vi "thermo_close.vi"(8 "error in":errorcluster, 11 "thermo in":T1={"type"=enum."COMET Tx5xx (ethernet)", "comment"="", "tag"="", "refresh"=0.0, "IP"="", "port"=0, "VISA"="", "last readout"=timestamp(0 s since 1904-01-01), "TCP ref"=refnum, "VISA sess"="", "idn"="", "press"=0.0, "RH"=0.0, "temp"=0.0, "pres cor"=[], "RH cor"=[], "temp cor"=[], "try left"=0, "failed"=FALSE, "RTD set"=[], "RTD inv"=[], "range"=0.0, "net mode"=enum."MODBUS", "try fail"=enum."Stop trying - return NaN", "timeout [s]"=0.0, "max retries"=0, "sim t [deg]"=0.0} {"RTD inv" format="%.1f"; "RTD set" format="%.1f"; "temp cor" format="%.1f"; "RH cor" format="%.1f"; "pres cor" format="%.1f"; "refresh" min=0.1 max=1000.0 format="%.2f"}) -> (0 "error out":errorcluster, 3 "thermo out":T1={"type"=enum."COMET Tx5xx (ethernet)", "comment"="", "tag"="", "refresh"=0.0, "IP"="", "port"=0, "VISA"="", "last readout"=timestamp(0 s since 1904-01-01), "TCP ref"=refnum, "VISA sess"="", "idn"="", "press"=0.0, "RH"=0.0, "temp"=0.0, "pres cor"=[], "RH cor"=[], "temp cor"=[], "try left"=0, "failed"=FALSE, "RTD set"=[], "RTD inv"=[], "range"=0.0, "net mode"=enum."MODBUS", "try fail"=enum."Stop trying - return NaN", "timeout [s]"=0.0, "max retries"=0, "sim t [deg]"=0.0} {"RTD inv" format="%.1f"; "RTD set" format="%.1f"; "temp cor" format="%.1f"; "RH cor" format="%.1f"; "pres cor" format="%.1f"; "refresh" min=0.1 max=1000.0 format="%.2f"})   [LabVIEW 2020]
uses:
  thermo.ctl
  thermo_types.ctl
  Thermometer Fail Action.ctl
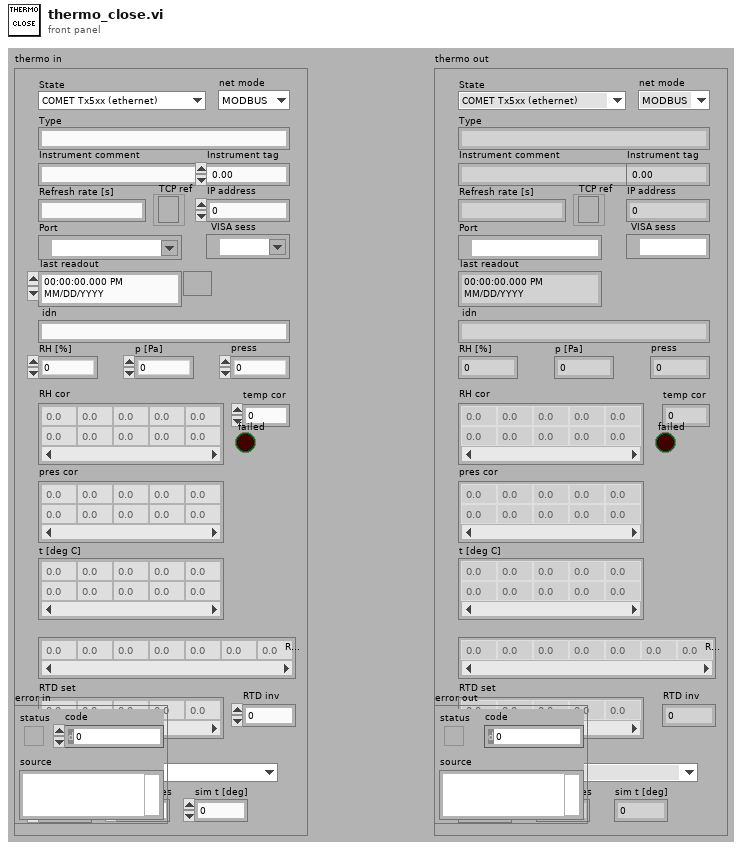
[diagram p1: front panel]
types:
  T1 = typedef "thermo.ctl" = cluster{"type":T2, "comment":string, "tag":string, "refresh":dbl, "IP":string, "port":u16, "VISA":refnum<visa-resource-name>, "last readout":timestamp, "TCP ref":refnum<k5>, "VISA sess":refnum<visa-resource-name>, "idn":string, "press":dbl, "RH":dbl, "temp":dbl, "pres cor":dbl[][], "RH cor":dbl[][], "temp cor":dbl[][], "try left":i32, "failed":bool, "RTD set":dbl[], "RTD inv":dbl[], "range":dbl, "net mode":enum16{"MODBUS", "HTTP"}, "try fail":T3, "timeout [s]":dbl, "max retries":i32, "sim t [deg]":dbl}
  T2 = typedef "thermo_types.ctl" = enum16{"Disabled", "Simulated", "COMET Tx5xx (ethernet)", "Keithley 2002 (GPIB) + RTD", "Agilent 344xx (GPIB) + RTD"}
  T3 = typedef "Thermometer Fail Action.ctl" = enum16{"Stop trying - keep last value", "Stop trying - return NaN", "Generate error - stop sweep"}
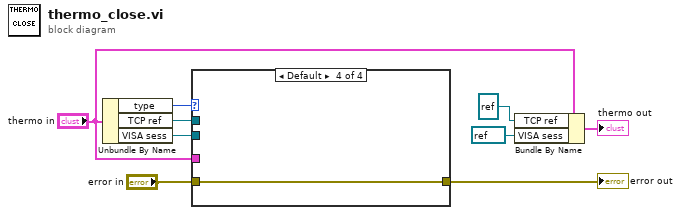
[diagram p0: block diagram]
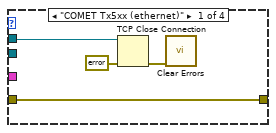
[diagram p2: hidden frame]
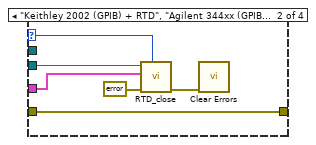
[diagram p3: hidden frame]
diagram:
  n1 = Unbundle By Name("thermo in") -> ("type"=w9:T2, "TCP ref"=w8:refnum<k5>, "VISA sess"=w7:refnum<visa-resource-name>)
  n2 = case shown="Default" w9 {
    selector: w9 -> [_ w15 _ _]
    tunnel: w8 -> [w12 _ _ _]
    tunnel: w7 -> [_ w17 _ _]
    tunnel: "error in" -> [w13 w19 w20 w21]
    tunnel: [w13 w19 w20 w21] -> w6
    tunnel: "thermo in" -> [_ w14 _ _]
    frame "COMET Tx5xx (ethernet)" {
      n3 = TCP Close Connection(connection ID=w12, error in (no error)=errorcluster {"status"=FALSE, "code"=0, "source"=""}) -> (error out=w11:errorcluster)  [unwired: 1 in, 1 out]
      n4 = call <vilib>:"Clear Errors.vi"("error in (no error)"=w11) -> ()  [unwired: 5 in, 2 out]
    }
    frame "Keithley 2002 (GPIB) + RTD", "Agilent 344xx (GPIB) + RTD" {
      n5 = call "RTD_close.vi"("type"=w15, "error in"=errorcluster {"status"=FALSE, "code"=0, "source"=""} ("error in (no error)"), "thermo channel"=w14, "VISA in"=w17) -> ("error out"=w16:errorcluster)  [unwired: 7 in]
      n6 = call <vilib>:"Clear Errors.vi"("error in (no error)"=w16) -> ()  [unwired: 5 in, 2 out]
    }
    frame "Simulated" {
    }
    frame Default {
    }
  }
  "error out" <- w6
  n7 = Bundle By Name(cluster="thermo in", "TCP ref"=refnum<k5> refnum ("connection ID"), "VISA sess"=refnum<visa-resource-name> refnum) -> (→"thermo out":T1)
